vi "4.- Prueba 2 con VISA.vi"() -> ()   [LabVIEW 2019]
uses:
  Controles/Amp_Frec.ctl
  <vilib>/Utility/error.llb/DialogType.ctl
  QMH_Support/Enqueue Message (Single).vi
  <vilib>/Utility/error.llb/Error Cluster From Error Code.vi
  <vilib>/ErrorRing/Error Ring.xnode
  QMH_Support/Message Queue.lvlib
  QMH_Support/User Event - Stop/User Event - Stop.lvlib
  DS360/DS360.lvlib
  K2002/K2002.lvlib
  CNT90/CNT90.lvlib
panel:
  in  "CNT90":refnum<visa-resource-name>
  in  "K2002":refnum<visa-resource-name>
  in  "DS360":refnum<visa-resource-name>
  out "mouse up?":bool
  out "EHL":i32
  out "# elements in queue":i32
  out "MHL":i32
  out "Instrumentos":i32
  in  "go_A":bool
  out "Voltaje a generar":dbl(knob) scale=0.0..10.0
  out "error out":errorcluster
  in  "stop":bool
  in  "generar":bool
  in  "Voltaje a Generar":dbl(slide)=7.0649350649350655 scale=0.0..10.0
  out "voltMon":dbl format="%.2f"
  out "frecMon":dbl format="%.2f"
  # "Ensayo Eléctrico Ponderación A"
  # "Monitoreo"
  # "Frecuencia"
  # "Hz"
  # "Voltaje"
  # "mV"
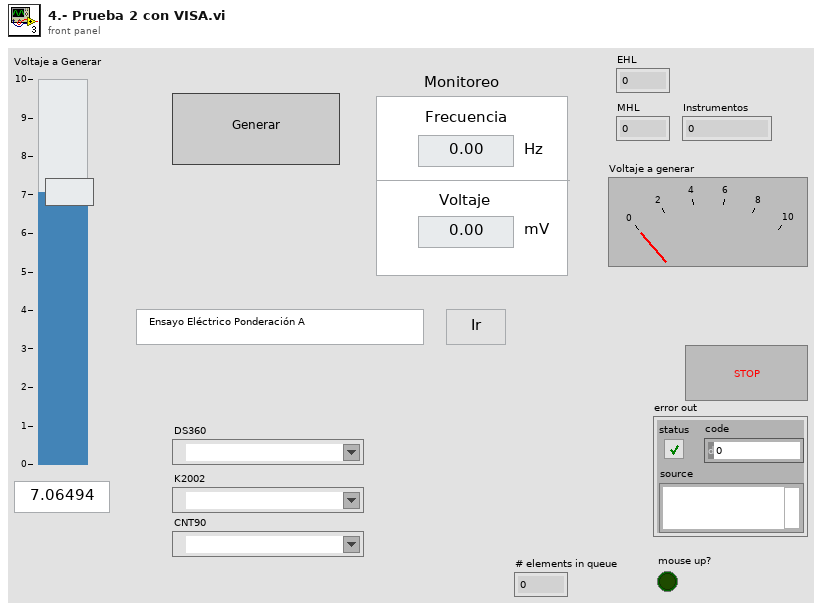
[diagram p1: front panel]
types:
  T1 = cluster{"DS360":refnum<visa-resource-name>, "K2002":refnum<visa-resource-name>, "CNT90":refnum<visa-resource-name>}
  T2 = typedef "Message Queue.lvlib/All Message Queues.ctl" = cluster{"MHL":refnum<queue>, "DS360":refnum<queue>, "K2002":refnum<queue>, "CNT90":refnum<queue>, "Instrumentos":refnum<queue>}
  T3 = typedef "Amp_Frec.ctl" = cluster{"Ampl":dbl, "Frec":dbl}
  T4 = typedef "DialogType.ctl" = u16
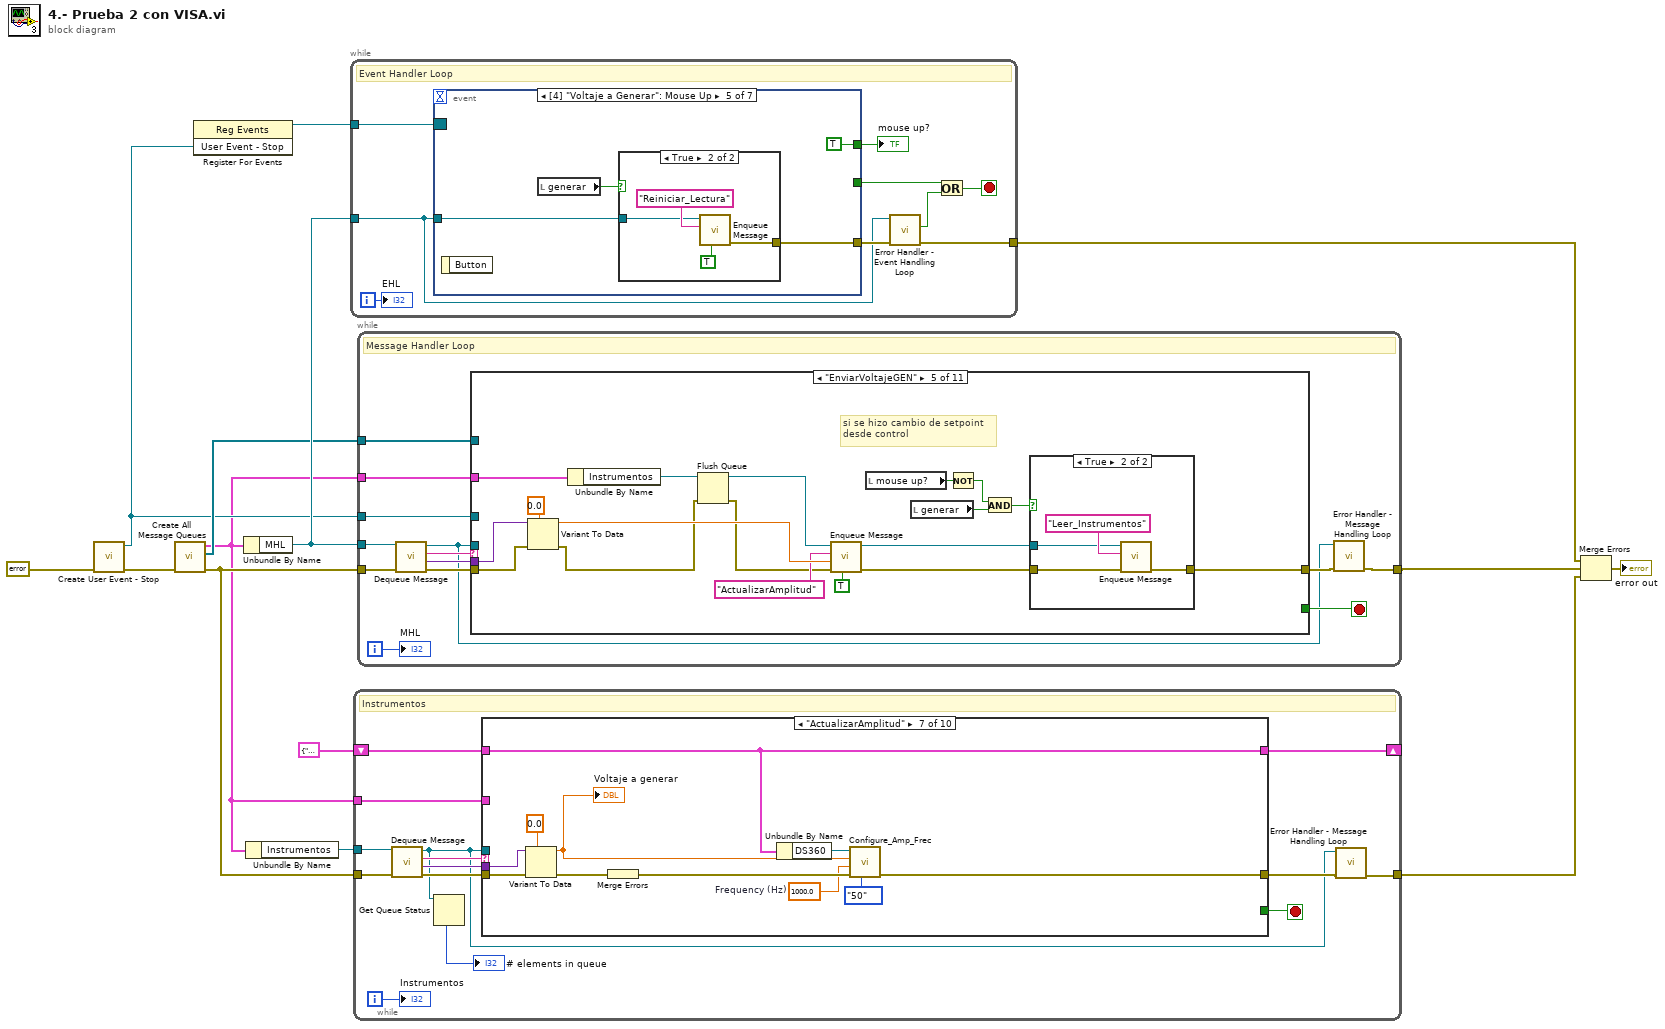
[diagram p0: block diagram]
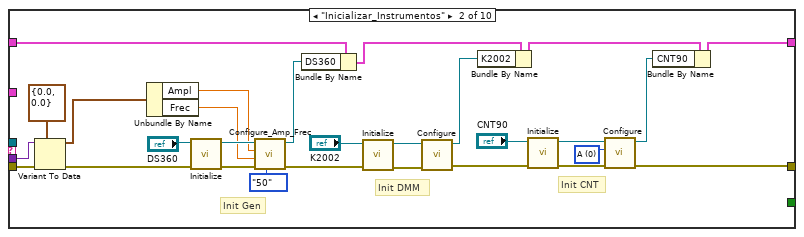
[diagram p3: hidden frame]
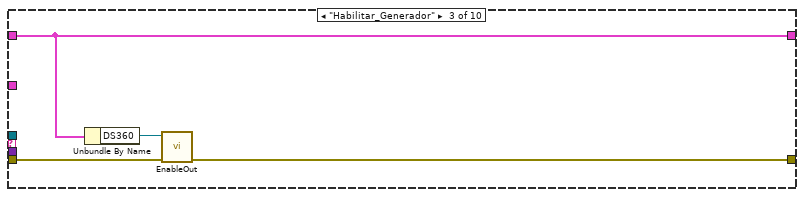
[diagram p4: hidden frame]
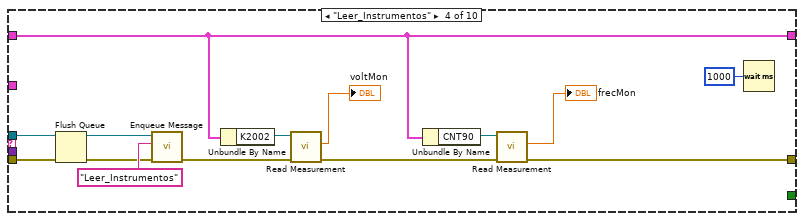
[diagram p5: hidden frame]
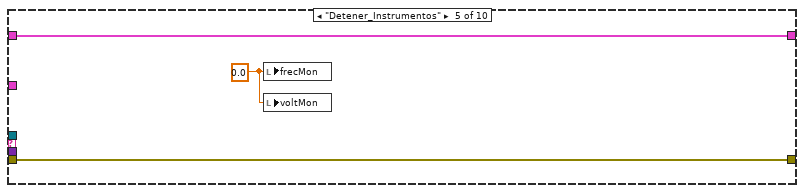
[diagram p6: hidden frame]
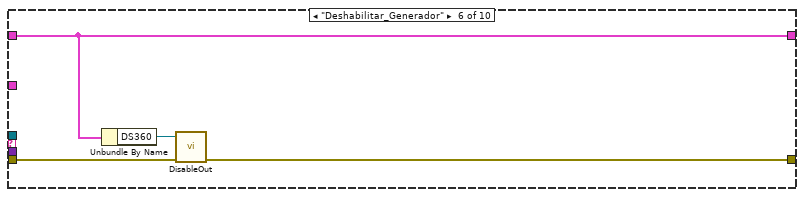
[diagram p7: hidden frame]
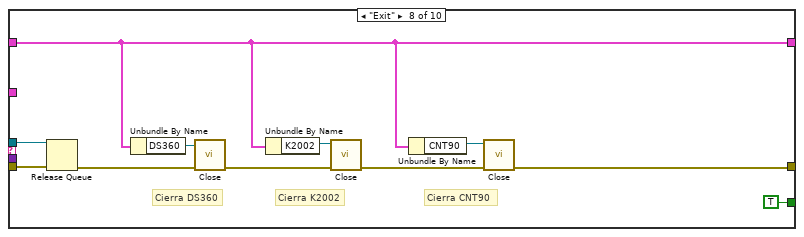
[diagram p8: hidden frame]
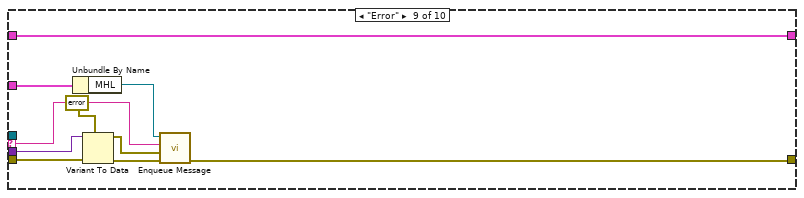
[diagram p9: hidden frame]
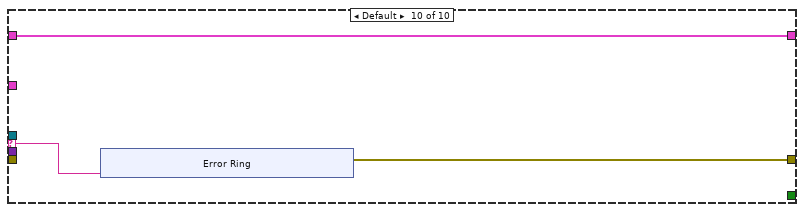
[diagram p10: hidden frame]
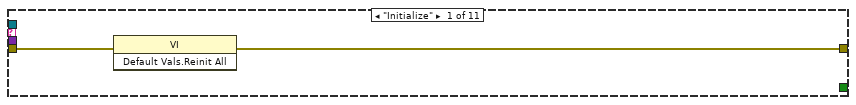
[diagram p11: hidden frame]
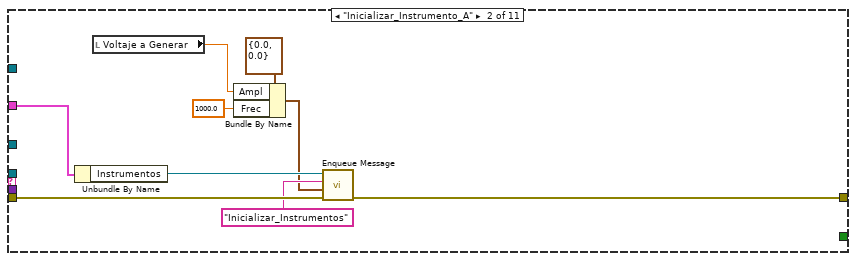
[diagram p12: hidden frame]
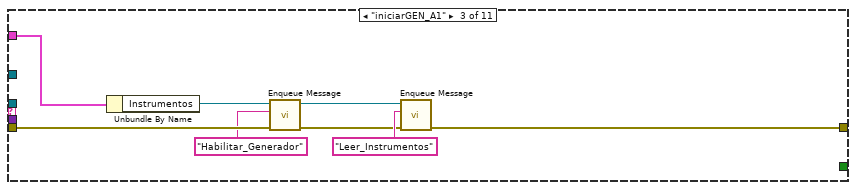
[diagram p13: hidden frame]
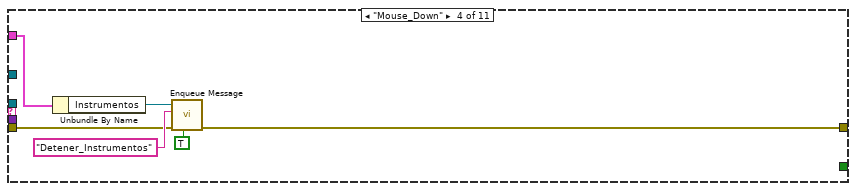
[diagram p14: hidden frame]
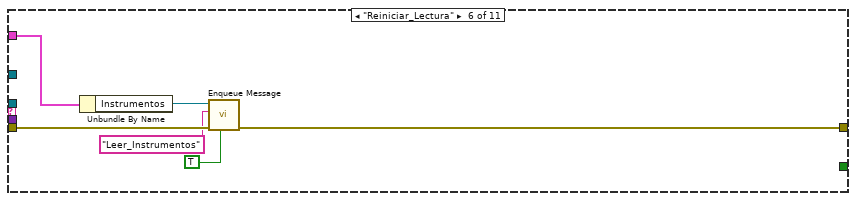
[diagram p16: hidden frame]
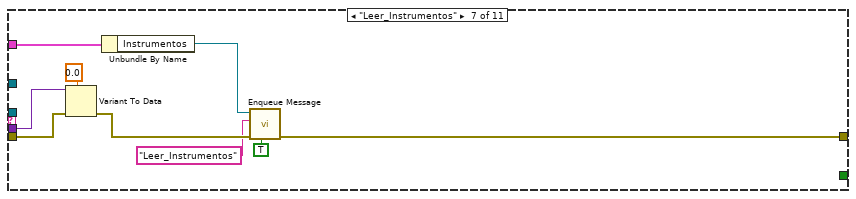
[diagram p17: hidden frame]
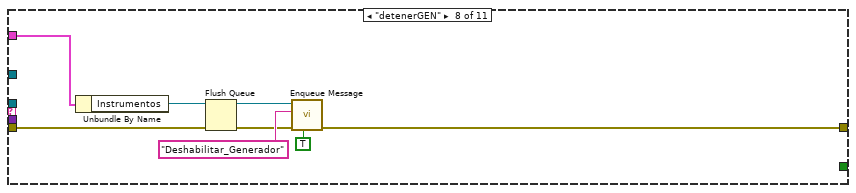
[diagram p18: hidden frame]
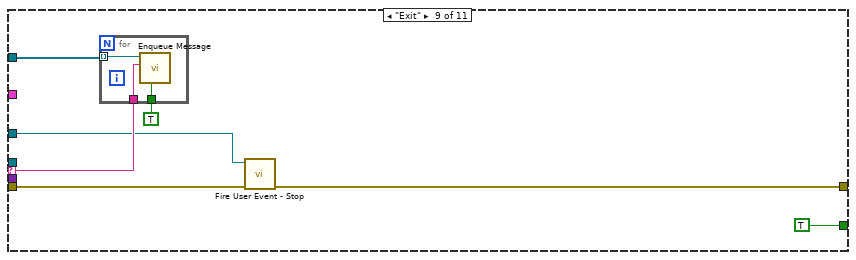
[diagram p19: hidden frame]
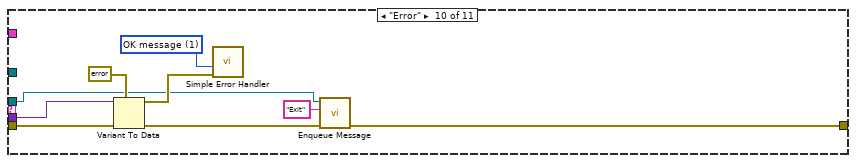
[diagram p20: hidden frame]
diagram:
  n1 = call "Create User Event - Stop.vi"("error in (no error)"=errorcluster {"status"=FALSE, "code"=0, "source"=""}) -> ("error out"=w8:errorcluster, "User Event - Stop"=w7:refnum<user-event>)  [unwired: 9 in]
  n2 = call "Create All Message Queues.vi"("error in (no error)"=w8) -> ("error out"=w4:errorcluster, "Queues Array"=w10:refnum<queue>[], "Message Queues out"=w2:T2)  [unwired: 8 in]
  n3 = register-events(w7) -> (reference out=w6:refnum<event-registration>)  [unwired: 2 in, 1 out]
  n4 = Unbundle By Name(w2) -> ("MHL"=w14:refnum<queue>)
  n5 = Unbundle By Name(w2) -> ("Instrumentos"=w5:refnum<queue>)
  n6 = while {
    tunnel: w14 -> [w20]
    tunnel: [w21] -> w13
    tunnel: w6 -> [w23]
    i -> [w16]
    stop <- w17 stop-if-true
    # "Event Handler Loop"
    n7 = event shown="[4] \"Voltaje a Generar\": Mouse Up" {
      selector: w23 -> [_ _ _ _ _ _ _]
      dyn-events: _ -> [_ _ _ _ _ _ _]
      timeout: _ -> [_ _ _ _ _ _ _]
      tunnel: w20 -> [w25 w28 w37 w43 w48 w57 _]
      tunnel: [w24 w27 w38 w42 w49 w55 _] -> w22
      tunnel: [_ _ _ _ _ _ TRUE] -> w19
      tunnel: [_ _ _ _ TRUE ("mouse up?") _ _] -> w15
      event "go_A": Value Change {
        n8 = event-data() -> ()  [unwired: 1 in, 1 out]
        n9 = call-poly "Enqueue Message.vi"("Message"="Inicializar_Instrumento_A" ("message"), "Message Queue"=w25) -> ("error out"=w24:errorcluster)  [unwired: 8 in, 1 out]
      }
      event "generar": Value Change {
        n10 = event-data() -> ("NewVal"=w29:bool)  [unwired: 1 in]
        n11 = Flush Queue(queue=w28) -> (queue out=w30:refnum<queue>, error out=w31:errorcluster)  [unwired: 1 in, 1 out]
        n12 = Select(t="iniciarGEN_A1" ("message"), s=w29, f="detenerGEN" ("message")) -> (s? t:f=w34:string)
        n13 = call-poly "Enqueue Message.vi"("Priority Message? (F)"=TRUE, "error in (no error)"=w31, "Message Data"="A1" ("message"), "Message"=w34, "Message Queue"=w30) -> ("error out"=w27:errorcluster)  [unwired: 5 in, 1 out]
      }
      event "Voltaje a Generar": Mouse Down {
        n14 = event-data() -> ()  [unwired: 1 in, 1 out]
        n15 = call-poly "Enqueue Message.vi"("Priority Message? (F)"=TRUE, "Message"="Mouse_Down" ("message"), "Message Queue"=w37) -> ("error out"=w38:errorcluster)  [unwired: 7 in, 1 out]
      }
      event "Voltaje a Generar": Value Change {
        n16 = event-data() -> ("NewVal"=w41:dbl)  [unwired: 1 in]
        n17 = call-poly "Enqueue Message.vi"("Priority Message? (F)"=TRUE, "Message Data"=w41, "Message"="EnviarVoltajeGEN" ("message"), "Message Queue"=w43) -> ("error out"=w42:errorcluster)  [unwired: 6 in, 1 out]
      }
      event "Voltaje a Generar": Mouse Up {
        n18 = event-data() -> ()  [unwired: 1 in, 1 out]
        n19 = local read "generar"() -> (w47:bool)
        n20 = case shown="True" w47 {
          tunnel: w48 -> [_ w52]
          tunnel: [errorcluster {"status"=FALSE, "code"=0, "source"=""} ("error out") w51] -> w49
          frame False {
          }
          frame True {
            n21 = call-poly "Enqueue Message.vi"("Priority Message? (F)"=TRUE, "Message"="Reiniciar_Lectura" ("message"), "Message Queue"=w52) -> ("error out"=w51:errorcluster)  [unwired: 7 in, 1 out]
          }
        }
      }
      event "stop": Value Change {
        n22 = event-data() -> ()  [unwired: 1 in, 1 out]
        n23 = call-poly "Enqueue Message.vi"("Message"="Exit", "Message Queue"=w57) -> ("error out"=w55:errorcluster)  [unwired: 8 in, 1 out]
      }
      event User Event {
        n24 = event-data() -> ()  [unwired: 1 in, 1 out]
      }
    }
    "mouse up?" <- w15
    n25 = call "Error Handler - Event Handling Loop.vi"("error in (no error)"=w22, "Message Queue"=w20) -> ("dup error in"=w21:errorcluster, "Error?"=w18:bool)  [unwired: 7 in, 1 out]
    n26 = Or(x=w19, y=w18) -> (x .or. y?=w17:bool)
    "EHL" <- w16
  }
  n27 = while {
    tunnel: w5 -> [w72]
    tunnel: w4 -> [w71]
    tunnel: [w64] -> w3
    tunnel: w2 -> [w63]
    shift-right: [w59] -> _
    shift-left: T1 {"DS360"="", "K2002"="", "CNT90"=""} -> [w60]
    i -> [w66]
    stop <- w67 stop-if-true
    # "Instrumentos"
    n28 = call "Dequeue Message.vi"("error in (no error)"=w71, "Message Queue"=w72) -> ("error out"=w70:errorcluster, "Message Data"=w68:variant, "Message"=w69:string, "dup Message Queue"=w62:refnum<queue>)  [unwired: 6 in]
    n29 = Get Queue Status(queue=w62) -> (# elements in queue=→"# elements in queue":i32)  [unwired: 2 in, 7 out]
    n30 = case shown="\"ActualizarAmplitud\"" w69 {
      selector: w69 -> [_ _ _ _ _ _ _ _ w154 w162]
      tunnel: w70 -> [w74 w102 w106 w118 w123 w127 w133 w149 w156 _]
      tunnel: w68 -> [_ w100 _ _ _ _ w137 _ w155 _]
      tunnel: w62 -> [_ _ _ w112 _ _ _ w148 _ _]
      tunnel: [w74 w76 w105 w117 w123 w126 w135 w146 w153 w161] -> w65
      tunnel: [_ _ _ _ _ _ _ TRUE _ _] -> w67
      tunnel: w63 -> [_ _ _ _ _ _ _ _ w152 _]
      tunnel: w60 -> [w73 w92 w103 w107 w121 w124 w129 w139 w150 w160]
      tunnel: [w73 w78 w103 w107 w121 w124 w129 w139 w150 w160] -> w59
      frame "Initialize" {
      }
      frame "Inicializar_Instrumentos" {
        w85 = 0 items=["A", "B"] ("Channel  1")
        # "Init CNT"
        # "Init DMM"
        # "Init Gen"
        n31 = Variant To Data(error in=w102, type=T3 {"Ampl"=0.0, "Frec"=0.0}, Variant=w100) -> (data=w99:T3, error out=w97:errorcluster)
        n32 = Unbundle By Name(w99) -> ("Ampl"=w94:dbl, "Frec"=w93:dbl)
        n33 = call "Initialize.vi"("error in (no error)"=w97, "VISA resource name"="DS360") -> ("error out"=w96:errorcluster, "VISA resource name out"=w95:refnum<visa-resource-name>)  [unwired: 8 in]
        n34 = call "Configure_Amp_Frec.vi"("Impedancia"=enum16{"50", "600", "HiZ"}."50", "error in (no error)"=w96, "Frequency (Hz)"=w93, "Amplitude (Vrms)"=w94, "VISA resource name"=w95) -> ("error out"=w89:errorcluster, "VISA resource name out"=w91:refnum<visa-resource-name>)  [unwired: 5 in]
        n35 = Bundle By Name(cluster=w92, "DS360"=w91) -> (w90:T1)
        n36 = call "Initialize.vi"("error in (no error)"=w89, "VISA resource name"="K2002") -> ("error out"=w87:errorcluster, "VISA resource name out"=w86:refnum<visa-resource-name>)  [unwired: 8 in]
        n37 = call "Configure.vi"("error in (no error)"=w87, "VISA resource name"=w86) -> ("error out"=w84:errorcluster, "VISA resource name out"=w80:refnum<visa-resource-name>)  [unwired: 8 in]
        n38 = Bundle By Name(cluster=w90, "K2002"=w80) -> (w81:T1)
        n39 = call "Initialize.vi"("error in (no error)"=w84, "VISA resource name"="CNT90") -> ("error out"=w83:errorcluster, "VISA resource name out"=w79:refnum<visa-resource-name>)  [unwired: 8 in]
        n40 = call "Configure.vi"("error in (no error)"=w83, "Channel  1"=w85, "VISA resource name"=w79) -> ("error out"=w76:errorcluster, "VISA resource name out"=w77:refnum<visa-resource-name>)  [unwired: 7 in]
        n41 = Bundle By Name(cluster=w81, "CNT90"=w77) -> (w78:T1)
      }
      frame "Habilitar_Generador" {
        n42 = Unbundle By Name(w103) -> ("DS360"=w104:refnum<visa-resource-name>)
        n43 = call "EnableOut.vi"("error in (no error)"=w106, "VISA resource name"=w104) -> ("error out"=w105:errorcluster)  [unwired: 8 in, 1 out]
      }
      frame "Leer_Instrumentos" {
        n44 = Flush Queue(queue=w112, error in (no error)=w118) -> (queue out=w111:refnum<queue>, error out=w113:errorcluster)  [unwired: 1 out]
        n45 = call-poly "Enqueue Message.vi"("error in (no error)"=w113, "Message"="Leer_Instrumentos", "Message Queue"=w111) -> ("error out"=w119:errorcluster)  [unwired: 7 in, 1 out]
        n46 = Unbundle By Name(w107) -> ("K2002"=w109:refnum<visa-resource-name>)
        n47 = call "Read Measurement.vi"("error in (no error)"=w119, "VISA resource name"=w109) -> ("error out"=w110:errorcluster, "Measurement"=→"voltMon":dbl)  [unwired: 7 in, 1 out]
        n48 = Unbundle By Name(w107) -> ("CNT90"=w108:refnum<visa-resource-name>)
        n49 = call "Read Measurement.vi"("error in (no error)"=w110, "VISA resource name"=w108) -> ("error out"=w117:errorcluster, "Measurement"=→"frecMon":dbl)  [unwired: 7 in, 1 out]
        n50 = Wait (ms)(milliseconds to wait=u32 1000) -> ()  [unwired: 1 out]
      }
      frame "Detener_Instrumentos" {
        w122 = 0.0 ("frecMon")
        n51 = local write "frecMon"(w122) -> ()
        n52 = local write "voltMon"(w122) -> ()
      }
      frame "Deshabilitar_Generador" {
        n53 = Unbundle By Name(w124) -> ("DS360"=w125:refnum<visa-resource-name>)
        n54 = call "DisableOut.vi"("error in (no error)"=w127, "VISA resource name"=w125) -> ("error out"=w126:errorcluster)  [unwired: 8 in, 1 out]
      }
      frame "ActualizarAmplitud" {
        w131 = 1000.0  # Frequency (Hz)
        n55 = Variant To Data(error in=w133, type=0.0, Variant=w137) -> (data=w134:dbl, error out=w136:errorcluster)
        "Voltaje a generar" <- w134
        n56 = Merge Errors(w136) -> (w132:errorcluster)
        n57 = Unbundle By Name(w129) -> ("DS360"=w130:refnum<visa-resource-name>)
        n58 = call "Configure_Amp_Frec.vi"("Impedancia"=enum16{"50", "600", "HiZ"}."50", "error in (no error)"=w132, "Frequency (Hz)"=w131, "Amplitude (Vrms)"=w134, "VISA resource name"=w130) -> ("error out"=w135:errorcluster)  [unwired: 5 in, 1 out]
      }
      frame "Exit" {
        # "Cierra CNT90"
        # "Cierra K2002"
        # "Cierra DS360"
        n59 = Release Queue(queue=w148, error in (no error)=w149) -> (error out=w142:errorcluster)  [unwired: 1 in, 2 out]
        n60 = Unbundle By Name(w139) -> ("DS360"=w140:refnum<visa-resource-name>)
        n61 = call "Close.vi"("error in (no error)"=w142, "VISA resource name"=w140) -> ("error out"=w141:errorcluster)  [unwired: 9 in]
        n62 = Unbundle By Name(w139) -> ("K2002"=w144:refnum<visa-resource-name>)
        n63 = call "Close.vi"("error in (no error)"=w141, "VISA resource name"=w144) -> ("error out"=w145:errorcluster)  [unwired: 9 in]
        n64 = Unbundle By Name(w139) -> ("CNT90"=w143:refnum<visa-resource-name>)
        n65 = call "Close.vi"("error in (no error)"=w145, "VISA resource name"=w143) -> ("error out"=w146:errorcluster)  [unwired: 9 in]
      }
      frame "Error" {
        n66 = Unbundle By Name(w152) -> ("MHL"=w151:refnum<queue>)
        n67 = Variant To Data(error in=w156, type=errorcluster {"status"=FALSE, "code"=0, "source"=""} ("error constant"), Variant=w155) -> (data=w157:errorcluster, error out=w158:errorcluster)
        n68 = call-poly "Enqueue Message.vi"("error in (no error)"=w158, "Message Data"=w157, "Message"=w154, "Message Queue"=w151) -> ("error out"=w153:errorcluster)  [unwired: 6 in, 1 out]
      }
      frame Default {
        n69 = xnode "Error Ring"("parameter 0"=w162) -> ("error out"=w161:errorcluster)
      }
    }
    n70 = call "Error Handler - Message Handling Loop.vi"("error in (no error)"=w65, "Message Queue"=w62) -> ("dup error in"=w64:errorcluster)  [unwired: 8 in, 1 out]
    "Instrumentos" <- w66
  }
  n71 = while {
    tunnel: w14 -> [w182]
    tunnel: w4 -> [w181]
    tunnel: [w173] -> w12
    tunnel: w10 -> [w177]
    tunnel: w7 -> [w175]
    tunnel: w2 -> [w171]
    i -> [w170]
    stop <- w176 stop-if-true
    # "Message Handler Loop"
    n72 = call "Dequeue Message.vi"("error in (no error)"=w181, "Message Queue"=w182) -> ("error out"=w178:errorcluster, "Message Data"=w179:variant, "Message"=w180:string, "dup Message Queue"=w172:refnum<queue>)  [unwired: 6 in]
    n73 = case shown="\"EnviarVoltajeGEN\"" w180 {
      selector: w180 -> [_ _ _ _ _ _ _ _ w259 _ w274]
      tunnel: w179 -> [_ _ _ _ w223 _ w243 _ _ w264 _]
      tunnel: w178 -> [w184 w192 w201 w204 w224 w236 w244 w252 w256 w267 _]
      tunnel: w172 -> [_ _ _ _ _ _ _ _ _ w265 _]
      tunnel: [w183 w193 w195 w207 w213 w232 w240 w250 w255 w266 w273] -> w174
      tunnel: w177 -> [_ _ _ _ _ _ _ _ w260 _ _]
      tunnel: [_ _ _ _ _ _ _ _ TRUE _ _] -> w176
      tunnel: w175 -> [_ _ _ _ _ _ _ _ w254 _ _]
      tunnel: w171 -> [_ w190 w200 w203 w222 w235 w242 w251 _ _ _]
      frame "Initialize" {
        n74 = invoke class="VI" method="Default Vals.Reinit All"(error in=w184) -> (error out=w183:errorcluster)  [unwired: 2 in, 2 out]
      }
      frame "Inicializar_Instrumento_A" {
        n75 = Unbundle By Name(w190) -> ("Instrumentos"=w189:refnum<queue>)
        n76 = local read "Voltaje a Generar"() -> (w186:dbl)
        n77 = Bundle By Name(cluster=T3 {"Ampl"=0.0, "Frec"=0.0}, "Ampl"=w186, "Frec"=1000.0) -> (w187:T3)
        n78 = call-poly "Enqueue Message.vi"("error in (no error)"=w192, "Message Data"=w187, "Message"="Inicializar_Instrumentos", "Message Queue"=w189) -> ("error out"=w193:errorcluster)  [unwired: 6 in, 1 out]
      }
      frame "iniciarGEN_A1" {
        n79 = Unbundle By Name(w200) -> ("Instrumentos"=w199:refnum<queue>)
        n80 = call-poly "Enqueue Message.vi"("error in (no error)"=w201, "Message"="Habilitar_Generador", "Message Queue"=w199) -> ("error out"=w196:errorcluster, "dup Message Queue"=w194:refnum<queue>)  [unwired: 7 in]
        n81 = call-poly "Enqueue Message.vi"("error in (no error)"=w196, "Message"="Leer_Instrumentos", "Message Queue"=w194) -> ("error out"=w195:errorcluster)  [unwired: 7 in, 1 out]
      }
      frame "Mouse_Down" {
        n82 = Unbundle By Name(w203) -> ("Instrumentos"=w202:refnum<queue>)
        n83 = call-poly "Enqueue Message.vi"("Priority Message? (F)"=TRUE, "error in (no error)"=w204, "Message"="Detener_Instrumentos", "Message Queue"=w202) -> ("error out"=w207:errorcluster)  [unwired: 6 in, 1 out]
      }
      frame "EnviarVoltajeGEN" {
        # "si se hizo cambio de setpoint\ndesde control"
        n84 = Variant To Data(error in=w224, type=0.0, Variant=w223) -> (data=w220:dbl, error out=w216:errorcluster)
        n85 = Unbundle By Name(w222) -> ("Instrumentos"=w221:refnum<queue>)
        n86 = Flush Queue(queue=w221, error in (no error)=w216) -> (queue out=w217:refnum<queue>, error out=w215:errorcluster)  [unwired: 1 out]
        n87 = call-poly "Enqueue Message.vi"("Priority Message? (F)"=TRUE, "error in (no error)"=w215, "Message Data"=w220, "Message"="ActualizarAmplitud", "Message Queue"=w217) -> ("error out"=w214:errorcluster, "dup Message Queue"=w212:refnum<queue>)  [unwired: 5 in]
        n88 = local read "mouse up?"() -> (w209:bool)
        n89 = local read "generar"() -> (w211:bool)
        n90 = Not(x=w209) -> (.not. x?=w208:bool)
        n91 = And(x=w208, y=w211) -> (x .and. y?=w210:bool)
        n92 = case shown="True" w210 {
          tunnel: w214 -> [w226 w229]
          tunnel: [w226 w228] -> w213
          tunnel: w212 -> [_ w227]
          frame False {
          }
          frame True {
            n93 = call-poly "Enqueue Message.vi"("error in (no error)"=w229, "Message"="Leer_Instrumentos" ("message"), "Message Queue"=w227) -> ("error out"=w228:errorcluster)  [unwired: 7 in, 1 out]
          }
        }
      }
      frame "Reiniciar_Lectura" {
        n94 = Unbundle By Name(w235) -> ("Instrumentos"=w234:refnum<queue>)
        n95 = call-poly "Enqueue Message.vi"("Priority Message? (F)"=TRUE, "error in (no error)"=w236, "Message"="Leer_Instrumentos", "Message Queue"=w234) -> ("error out"=w232:errorcluster)  [unwired: 6 in, 1 out]
      }
      frame "Leer_Instrumentos" {
        n96 = Variant To Data(error in=w244, type=0.0, Variant=w243) -> (error out=w241:errorcluster)  [unwired: 1 out]
        n97 = Unbundle By Name(w242) -> ("Instrumentos"=w237:refnum<queue>)
        n98 = call-poly "Enqueue Message.vi"("Priority Message? (F)"=TRUE, "error in (no error)"=w241, "Message"="Leer_Instrumentos", "Message Queue"=w237) -> ("error out"=w240:errorcluster)  [unwired: 6 in, 1 out]
      }
      frame "detenerGEN" {
        n99 = Unbundle By Name(w251) -> ("Instrumentos"=w247:refnum<queue>)
        n100 = Flush Queue(queue=w247, error in (no error)=w252) -> (queue out=w246:refnum<queue>, error out=w248:errorcluster)  [unwired: 1 out]
        n101 = call-poly "Enqueue Message.vi"("Priority Message? (F)"=TRUE, "error in (no error)"=w248, "Message"="Deshabilitar_Generador", "Message Queue"=w246) -> ("error out"=w250:errorcluster)  [unwired: 6 in, 1 out]
      }
      frame "Exit" {
        n102 = for {
          tunnel: w260 -> [w263] mode=indexing
          tunnel: w259 -> [w262]
          tunnel: TRUE -> [w261]
          n103 = call-poly "Enqueue Message.vi"("Priority Message? (F)"=w261, "Message"=w262, "Message Queue"=w263) -> ()  [unwired: 7 in, 2 out]
        }
        n104 = call "Fire User Event - Stop.vi"("error in (no error)"=w256, "User Event - Stop"=w254) -> ("error out"=w255:errorcluster)  [unwired: 9 in]
      }
      frame "Error" {
        w271 = T4 1 items=["no dialog", "OK message", "continue or stop message", "OK message + warnings", "continue/stop + warnings"] ("type of dialog (OK msg:1)")
        n105 = Variant To Data(error in=w267, type=errorcluster {"status"=FALSE, "code"=0, "source"=""} ("error out"), Variant=w264) -> (data=w269:errorcluster, error out=w268:errorcluster)
        n106 = call <vilib>:"Simple Error Handler.vi"("type of dialog (OK msg:1)"=w271, "error in (no error)"=w269) -> ()  [unwired: 3 in, 5 out]
        n107 = call-poly "Enqueue Message.vi"("error in (no error)"=w268, "Message"="Exit", "Message Queue"=w265) -> ("error out"=w266:errorcluster)  [unwired: 7 in, 1 out]
      }
      frame Default {
        n108 = xnode "Error Ring"("parameter 0"=w274) -> ("error out"=w273:errorcluster)
      }
    }
    n109 = call "Error Handler - Message Handling Loop.vi"("error in (no error)"=w174, "Message Queue"=w172) -> ("dup error in"=w173:errorcluster)  [unwired: 8 in, 1 out]
    "MHL" <- w170
  }
  n110 = Merge Errors(w13, w12, w3) -> (→"error out":errorcluster)
